vi "Config.vi"() -> ()   [LabVIEW 2020]
uses:
  Global_Variable/A131258.vi
  Database/Global1.vi
  Global_Variable/Global.vi
  <vilib>/Utility/config.llb/NI_LVConfig.lvlib
panel:
  in  "系数":bool
  in  "产品型号":string(combo)
  in  "删除":bool
  in  "确定":bool
  in  "添加":bool
  in  "退出":bool
  in  "更新":bool
  in  "选项卡控件":enum32{"产品参数", "系统参数"}(tab)
  in  "判定框范围":string[][](table)=[["°"], ["N"], ["°"], ["N"], ["°"], ["N"], ["°"], ["N"]]
  in  "工位坐标轴参数":string[][](table)=[["°"], ["N"], ["°"], ["N"], ["mm"], ["N"], ["mm"], ["N"]]
  in  "结果判定参数":string[][](table)=[["N"], ["N"], ["N"], ["N"], ["N"], ["N"], ["N"], ["N"], ["N"]]
  in  "工位滤波":cluster{"启用滤波":bool, "滤波系数":dbl}
  in  "系统参数设置":string[][](table)=[[""], [""], [""], [""]]
  # "磨合台"
types:
  T1 = enum8{"Enabled", "Disabled", "Disabled and Grayed Out"}
  T2 = typedef "NI_LVConfig.lvlib/Config Data RefNum.ctl" = refnum<k1>
  T3 = cluster{"用户编号":string, "用户名":string, "用户密码(密文)":string, "用户权限":string}
  T4 = cluster{"[0]":cluster{dbl, dbl}, "[1]":cluster{dbl, dbl}, "[2]":cluster{dbl, dbl}, "[3]":cluster{dbl, dbl}, "[4]":cluster{dbl, dbl}, "[5]":cluster{dbl, dbl}, "[6]":cluster{dbl, dbl}, "[7]":cluster{dbl, dbl}, "[8]":cluster{dbl, dbl}}
  T5 = cluster{"[0]":cluster{string, dbl, dbl}, "[1]":cluster{string, dbl, dbl}, "[2]":cluster{string, dbl, dbl}, "[3]":cluster{string, dbl, dbl}}
  T6 = cluster{"[0]":cluster{string, dbl, dbl}, "[1]":cluster{string, dbl, dbl}, "[2]":cluster{string, dbl, dbl}, "[3]":cluster{string, dbl, dbl}, "[4]":cluster{string, dbl, dbl}, "[5]":cluster{string, dbl, dbl}, "[6]":cluster{string, dbl, dbl}, "[7]":cluster{string, dbl, dbl}, "[8]":cluster{string, dbl, dbl}, "[9]":cluster{string, dbl, dbl}}
  T7 = cluster{"正向判定X值":cluster{"单位":string, "下限":dbl, "上限":dbl}, "正向判定Y值":cluster{"单位":string, "下限":dbl, "上限":dbl}, "逆向判定X值":cluster{"单位":string, "下限":dbl, "上限":dbl}, "逆向判定Y值":cluster{"单位":string, "下限":dbl, "上限":dbl}}
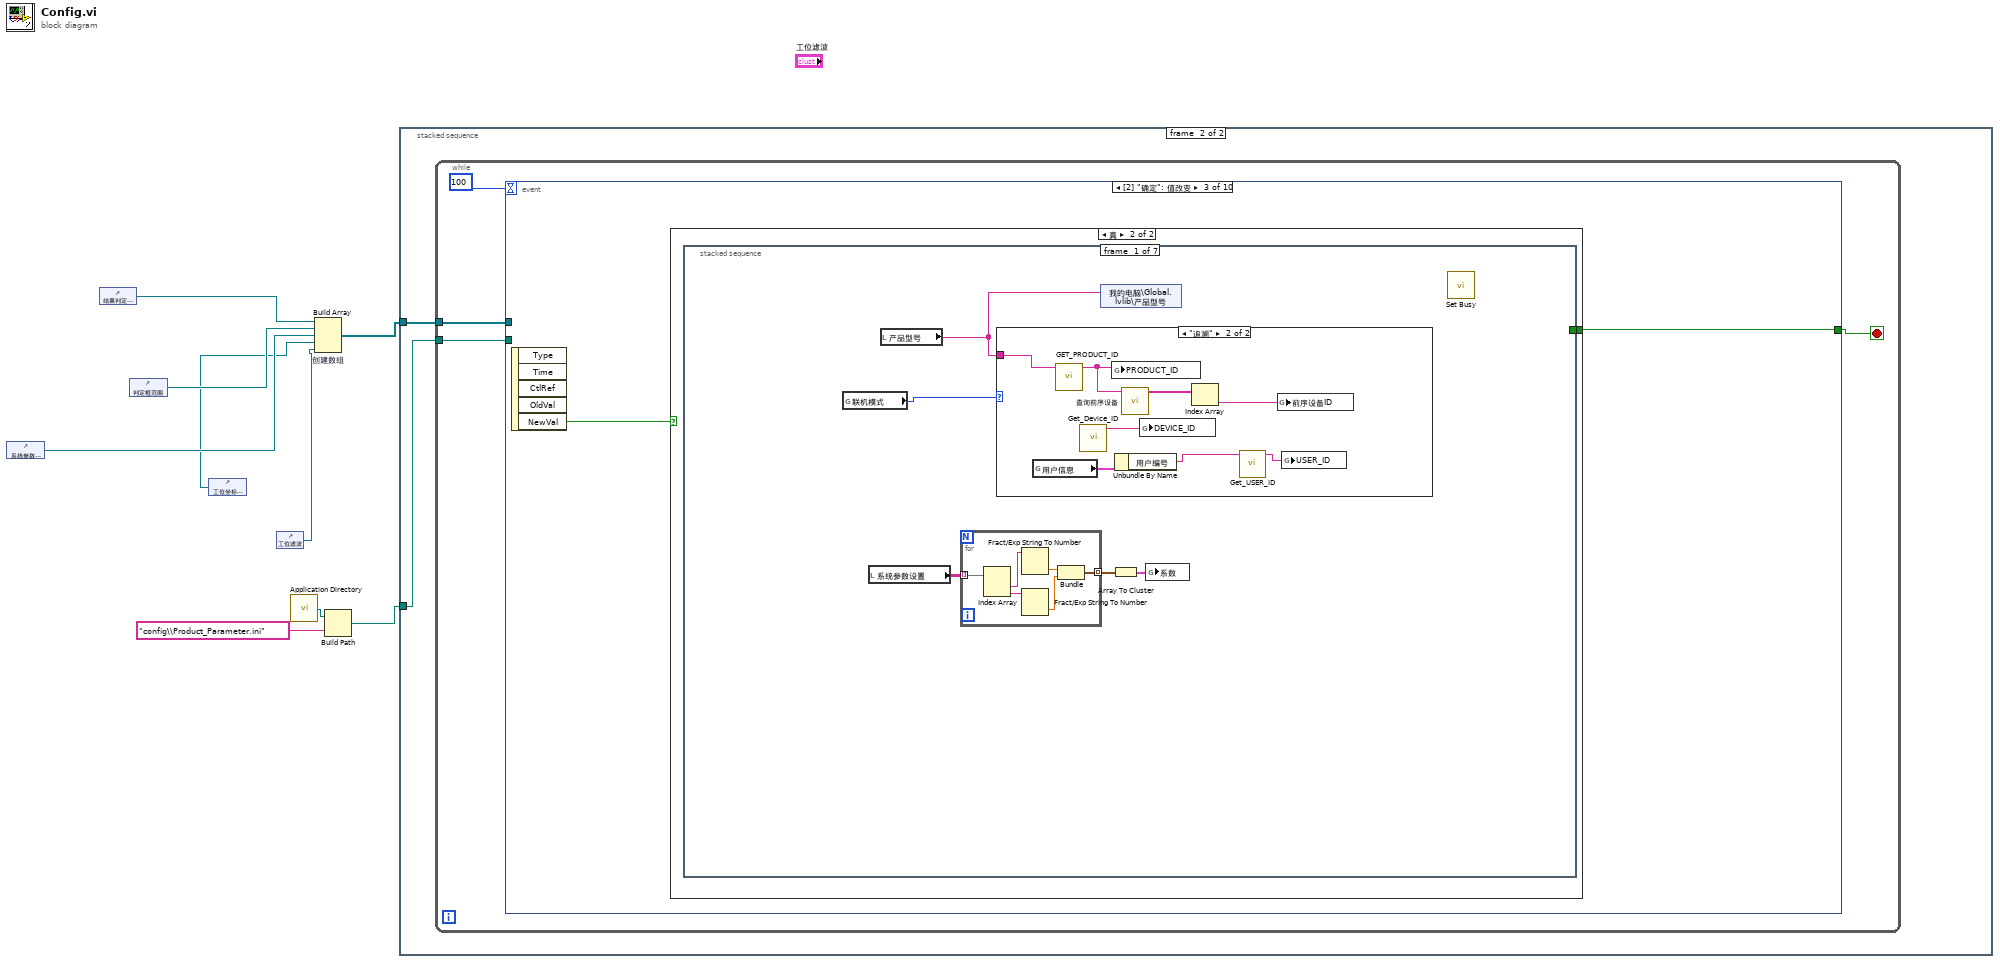
[diagram p0: block diagram]
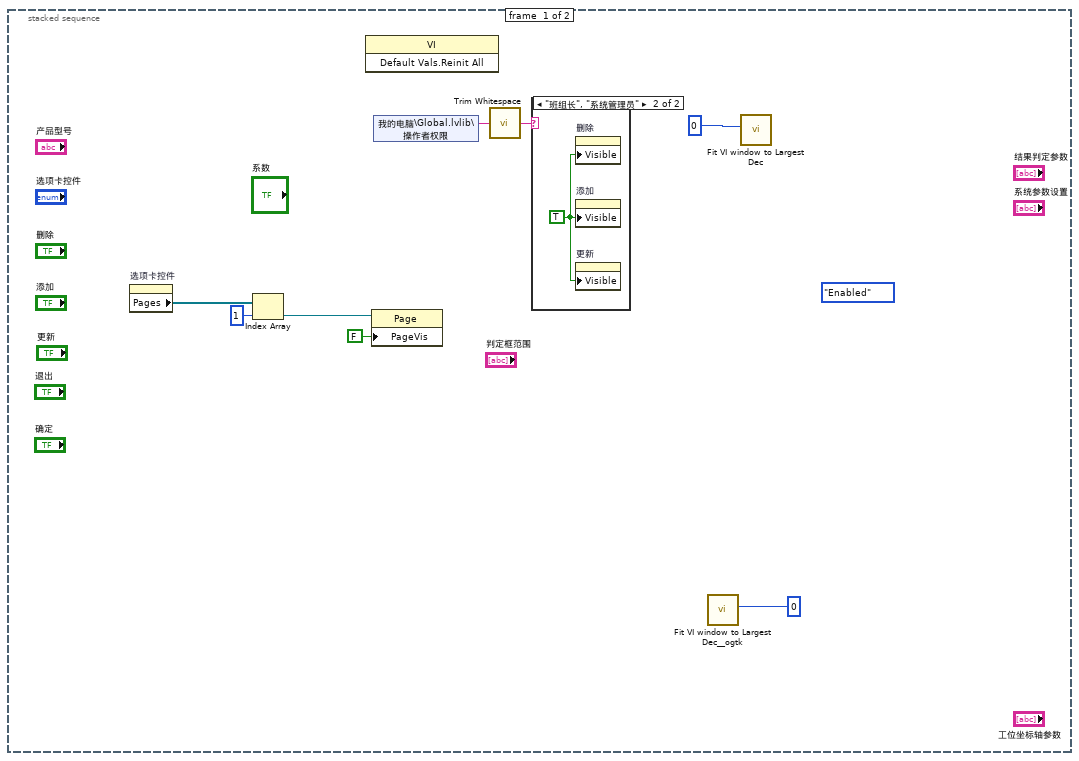
[diagram p2: hidden frame]
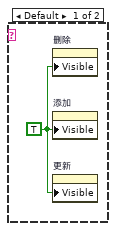
[diagram p3: hidden frame]
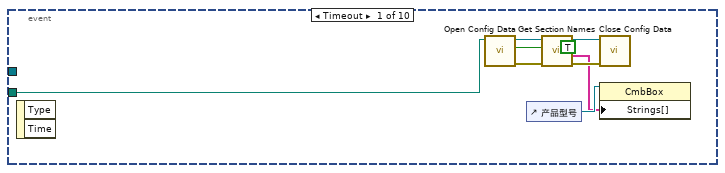
[diagram p4: hidden frame]
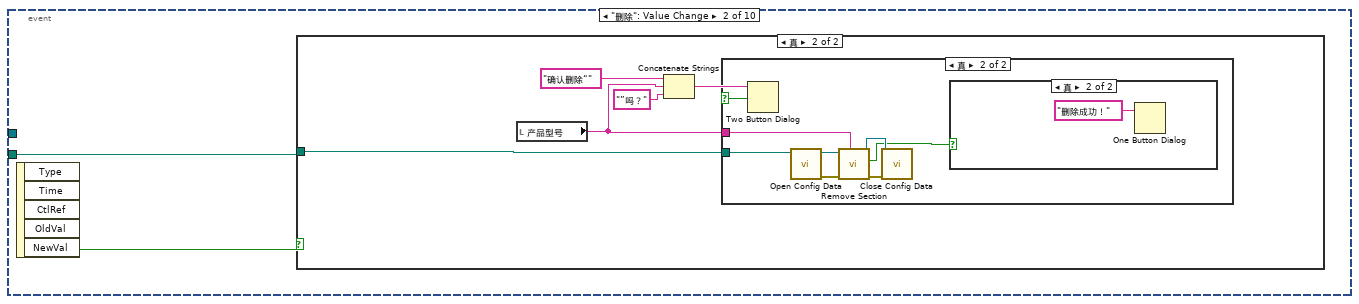
[diagram p5: hidden frame]
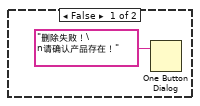
[diagram p8: hidden frame]
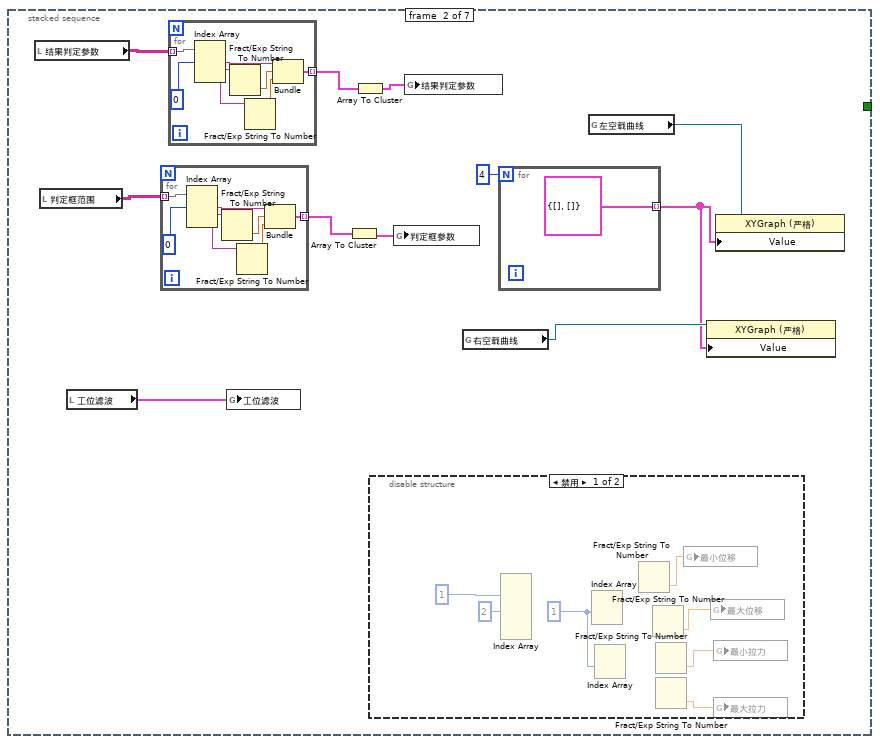
[diagram p11: hidden frame]
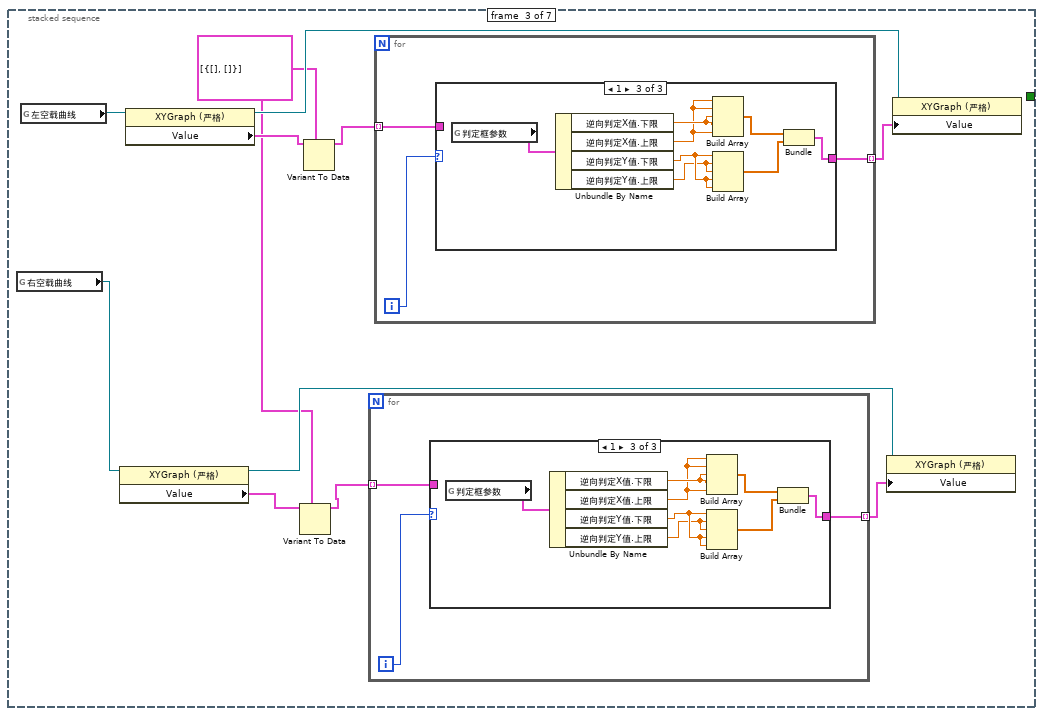
[diagram p13: hidden frame]
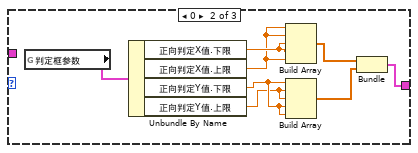
[diagram p15: hidden frame]
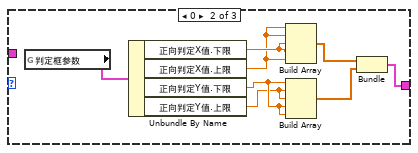
[diagram p17: hidden frame]
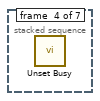
[diagram p18: hidden frame]
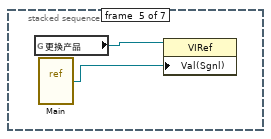
[diagram p19: hidden frame]
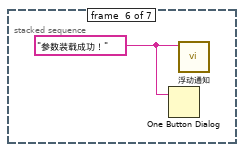
[diagram p20: hidden frame]
diagram:
  n1 = control-ref of="系统参数设置"() -> (w6:refnum<vi>)
  n2 = control-ref of="结果判定参数"() -> (w5:refnum<vi>)
  n3 = control-ref of="判定框范围"() -> (w3:refnum<vi>)
  n4 = control-ref of="工位坐标轴参数"() -> (w2:refnum<vi>)
  n5 = control-ref of="工位滤波"() -> (w1:refnum<vi>)
  n6 = call <vilib>:"Application Directory.vi"() -> ("Application Directory"=w8:path)
  n7 = Build Array "创建数组"(w5, w3, w6, w2, w1) -> (w9:refnum<vi>[])
  n8 = Build Path(base path=w8, name or relative path="config\\Product_Parameter.ini" ("名称或相对路径")) -> (appended path=w7:path)
  n9 = stacked-sequence {
    tunnel: w9 -> [_ w20]
    tunnel: w7 -> [_ w21]
    frame #0 {
      (unwired) T1."Enabled" ("禁用")
      n10 = property on="选项卡控件" class="TabCtl (严格)"() -> ("Pages"=w12:refnum<vi>[])  [unwired: 2 in, 2 out]
      n11 = Index Array(array=w12, index=1 ("索引")) -> (element=w13:refnum<vi>)
      n12 = invoke class="VI" method="Default Vals.Reinit All"() -> ()  [unwired: 3 in, 3 out]
      n13 = property class="Page"(reference=w13, "PageVis"=FALSE ("选项卡可见")) -> ()  [unwired: 1 in, 2 out]
      n14 = shared-variable "我的电脑\\Global.lvlib\\操作者权限"() -> (w17:string)  [unwired: 1 in, 1 out]
      n15 = call <vilib>:"Trim Whitespace.vi"("string"=w17) -> ("trimmed string"=w16:string)  [unwired: 1 in]
      n16 = case shown="\"班组长\", \"系统管理员\"" w16 {
        frame Default {
          w18 = TRUE ("可见")
          n17 = property on="删除" class="Bool (严格)"("Visible"=w18) -> ()  [unwired: 2 in, 2 out]
          n18 = property on="添加" class="Bool (严格)"("Visible"=w18) -> ()  [unwired: 2 in, 2 out]
          n19 = property on="更新" class="Bool (严格)"("Visible"=w18) -> ()  [unwired: 2 in, 2 out]
        }
        frame "班组长", "系统管理员" {
          w19 = TRUE ("可见")
          n20 = property on="删除" class="Bool (严格)"("Visible"=w19) -> ()  [unwired: 2 in, 2 out]
          n21 = property on="添加" class="Bool (严格)"("Visible"=w19) -> ()  [unwired: 2 in, 2 out]
          n22 = property on="更新" class="Bool (严格)"("Visible"=w19) -> ()  [unwired: 2 in, 2 out]
        }
      }
      n23 = call <userlib>:"Fit VI window to Largest Dec__ogtk.vi"("border spacing (2 px)"=0) -> ()  [unwired: 5 in, 2 out]
      n24 = call "Fit VI window to Largest Dec.vi"("border spacing (2 px)"=0) -> ()  [unwired: 5 in, 2 out]
    }
    frame #1 {
      n25 = while {
        tunnel: w21 -> [w25]
        tunnel: w20 -> [w22]
        stop <- w24 stop-if-true
        n26 = event shown="[2] \"确定\": 值改变" {
          selector: _ -> [_ _ _ _ _ _ _ _ _ _]
          dyn-events: _ -> [_ _ _ _ _ _ _ _ _ _]
          timeout: 100 -> [_ _ _ _ _ _ _ _ _ _]
          tunnel: w25 -> [w28 w35 _ w166 w194 _ w217 _ _ _]
          tunnel: [_ _ w51 _ _ TRUE _ _ _ TRUE] -> w24
          tunnel: w22 -> [_ _ _ w164 w192 _ w215 _ _ _]
          event Timeout {
            n27 = event-data() -> ()  [unwired: 1 in, 2 out]
            n28 = call <vilib>:"Open Config Data.vi"("create file if necessary (T)"=TRUE, "configuration file path"=w28) -> ("error out"=w30:errorcluster, "refnum"=w29:T2)  [unwired: 7 in, 1 out]
            n29 = control-ref of="产品型号"() -> (w27:refnum<vi>)
            n30 = call <vilib>:"Get Section Names.vi"("error in (no error)"=w30, "refnum"=w29) -> ("error out"=w32:errorcluster, "section names"=w26:string[], "refnum out"=w31:T2)  [unwired: 7 in]
            n31 = call <vilib>:"Close Config Data.vi"("error in (no error)"=w32, "refnum"=w31) -> ()  [unwired: 8 in, 2 out]
            n32 = property on="属性节点" class="CmbBox"(reference=w27, "Strings[]"=w26) -> ()  [unwired: 1 in, 2 out]
          }
          event "删除": Value Change {
            n33 = event-data() -> ("NewVal"=w34:bool)  [unwired: 1 in, 4 out]
            n34 = case shown="真" w34 {
              tunnel: w35 -> [_ w37]
              frame False {
              }
              frame True {
                n35 = local read "产品型号"() -> (w36:string)
                n36 = Concatenate Strings("确认删除“", w36, "”吗？") -> (w39:string)
                n37 = Two Button Dialog(message=w39) -> (T button?=w38:bool)  [unwired: 2 in]
                n38 = case shown="真" w38 {
                  tunnel: w37 -> [_ w43]
                  tunnel: w36 -> [_ w42]
                  frame False {
                  }
                  frame True {
                    n39 = call <vilib>:"Open Config Data.vi"("configuration file path"=w43) -> ("error out"=w45:errorcluster, "refnum"=w48:T2)  [unwired: 8 in, 1 out]
                    n40 = call <vilib>:"Remove Section.vi"("section"=w42, "error in (no error)"=w45, "refnum"=w48) -> ("error out"=w47:errorcluster, "section exists?"=w44:bool, "refnum out"=w46:T2)  [unwired: 6 in]
                    n41 = call <vilib>:"Close Config Data.vi"("error in (no error)"=w47, "refnum"=w46) -> ()  [unwired: 8 in, 2 out]
                    n42 = case shown="真" w44 {
                      frame False {
                        n43 = One Button Dialog(message="删除失败！\n请确认产品存在！" ("消息")) -> ()  [unwired: 1 in, 1 out]
                      }
                      frame True {
                        n44 = One Button Dialog(message="删除成功！" ("消息")) -> ()  [unwired: 1 in, 1 out]
                      }
                    }
                  }
                }
              }
            }
          }
          event "确定": Value Change {
            n45 = event-data() -> ("NewVal"=w52:bool)  [unwired: 1 in, 4 out]
            n46 = case shown="真" w52 {
              tunnel: [_ w53] -> w51
              frame False {
              }
              frame True {
                n47 = stacked-sequence {
                  tunnel: [_ _ _ _ _ _ TRUE] -> w53
                  frame #0 {
                    n48 = global read "Global1.vi" "联机模式"() -> (w57:enum16{"单机", "追溯"})
                    n49 = local read "系统参数设置"() -> (w56:string[][])
                    n50 = local read "产品型号"() -> (w58:string)
                    n51 = for {
                      tunnel: w56 -> [w64] mode=indexing
                      tunnel: [w61] -> w55 mode=indexing
                      n52 = Index Array(array=w64) -> (element #1=w60:string, element #2=w59:string)  [unwired: 2 in]
                      n53 = Fract/Exp String To Number(string=w60) -> (number=w63:dbl)  [unwired: 3 in, 1 out]
                      n54 = Fract/Exp String To Number(string=w59) -> (number=w62:dbl)  [unwired: 3 in, 1 out]
                      n55 = Bundle(w63, w62) -> (w61:cluster{dbl, dbl})  [unwired: 1 in]
                    }
                    n56 = case shown="\"追溯\"" w57 {
                      tunnel: w58 -> [_ w72]
                      frame "单机", Default {
                      }
                      frame "追溯" {
                        n57 = global read "Global1.vi" "用户信息"() -> (w67:T3)
                        n58 = call "GET_PRODUCT_ID.vi"("PRODFUCT_NAME"=w72) -> ("PRODUCT_ID"=w71:string)  [unwired: 10 in]
                        n59 = call "Get_Device_ID.vi"() -> ("Device_ID"=w68:string)  [unwired: 10 in, 1 out]
                        n60 = global write "追溯Global.vi" "PRODUCT_ID"(w71) -> ()
                        n61 = Unbundle By Name(w67) -> ("用户编号"=w66:string)
                        n62 = call "查询前序设备.vi"("PRODUCT_ID"=w71) -> ("前序工位"=w70:string[])  [unwired: 10 in]
                        n63 = global write "追溯Global.vi" "DEVICE_ID"(w68) -> ()
                        n64 = Index Array(array=w70) -> (element=w69:string)  [unwired: 1 in]
                        n65 = call "Get_USER_ID.vi"("USER_EMPLOYEE_ID"=w66) -> ("USER_ID"=w65:string)  [unwired: 9 in, 1 out]
                        n66 = global write "追溯Global.vi" "前序设备ID"(w69) -> ()
                        n67 = global write "追溯Global.vi" "USER_ID"(w65) -> ()
                      }
                    }
                    n68 = shared-variable "我的电脑\\Global.lvlib\\产品型号"(w58) -> ()  [unwired: 1 in, 1 out]
                    n69 = Array To Cluster(array=w55) -> (cluster=w54:T4)
                    n70 = global write "A131258.vi" "系数"(w54) -> ()
                    n71 = call <vilib>:"Set Busy.vi"() -> ()  [unwired: 10 in, 2 out]
                  }
                  frame #1 {
                    n72 = local read "结果判定参数"() -> (w82:string[][])
                    n73 = local read "判定框范围"() -> (w81:string[][])
                    n74 = local read "工位滤波"() -> (w73:cluster{"启用滤波":bool, "滤波系数":dbl})
                    n75 = for {
                      tunnel: w81 -> [w95] mode=indexing
                      tunnel: [w97] -> w80 mode=indexing
                      n76 = Index Array(array=w95, index #1=0) -> (element #1=w96:string, element #2=w94:string, element #3=w93:string)  [unwired: 2 in]
                      n77 = Fract/Exp String To Number(string=w94) -> (number=w99:dbl)  [unwired: 3 in, 1 out]
                      n78 = Fract/Exp String To Number(string=w93) -> (number=w98:dbl)  [unwired: 3 in, 1 out]
                      n79 = Bundle(w96, w99, w98) -> (w97:cluster{string, dbl, dbl})  [unwired: 1 in]
                    }
                    n80 = for {
                      tunnel: w82 -> [w103] mode=indexing
                      tunnel: [w105] -> w83 mode=indexing
                      n81 = Index Array(array=w103, index #1=0) -> (element #1=w104:string, element #2=w102:string, element #3=w101:string)  [unwired: 2 in]
                      n82 = Fract/Exp String To Number(string=w102) -> (number=w107:dbl)  [unwired: 3 in, 1 out]
                      n83 = Fract/Exp String To Number(string=w101) -> (number=w106:dbl)  [unwired: 3 in, 1 out]
                      n84 = Bundle(w104, w107, w106) -> (w105:cluster{string, dbl, dbl})  [unwired: 1 in]
                    }
                    n85 = global write "A131258.vi" "工位滤波"(w73) -> ()
                    n86 = Array To Cluster(array=w80) -> (cluster=w79:T5)
                    n87 = Array To Cluster(array=w83) -> (cluster=w78:T6)
                    n88 = disable-structure shown="禁用" {
                      frame Disabled {
                        w85 = 1 ("索引")
                        n89 = Index Array(index (row) #1=1 ("索引 (行)"), index (row) #2=2 ("索引 (行)")) -> ()  [unwired: 5 in, 3 out]
                        n90 = Index Array(index #1=w85) -> ()  [unwired: 2 in, 2 out]
                        n91 = Index Array(index #1=w85) -> ()  [unwired: 2 in, 2 out]
                        n92 = Fract/Exp String To Number() -> (number=w90:dbl)  [unwired: 4 in, 1 out]
                        n93 = Fract/Exp String To Number() -> (number=w89:dbl)  [unwired: 4 in, 1 out]
                        n94 = Fract/Exp String To Number() -> (number=w88:dbl)  [unwired: 4 in, 1 out]
                        n95 = Fract/Exp String To Number() -> (number=w87:dbl)  [unwired: 4 in, 1 out]
                        n96 = global write "判定参数.vi" "最小位移"(w90) -> ()
                        n97 = global write "判定参数.vi" "最大位移"(w89) -> ()
                        n98 = global write "判定参数.vi" "最小拉力"(w88) -> ()
                        n99 = global write "判定参数.vi" "最大拉力"(w87) -> ()
                      }
                      frame Enabled {
                      }
                    }
                    n100 = global write "A131258.vi" "判定框参数"(w79) -> ()
                    n101 = global write "A131258.vi" "结果判定参数"(w78) -> ()
                    n102 = global read "A131258.vi" "右空载曲线"() -> (w75:refnum<vi>)
                    n103 = for {
                      N: 4 -> [_]
                      tunnel: [cluster{dbl[], dbl[]} {[], []}] -> w74 mode=indexing
                    }
                    n104 = global read "A131258.vi" "左空载曲线"() -> (w77:refnum<vi>)
                    n105 = property class="XYGraph (严格)"(reference=w75, "Value"=w74) -> ()  [unwired: 1 in, 2 out]
                    n106 = property class="XYGraph (严格)"(reference=w77, "Value"=w74) -> ()  [unwired: 1 in, 2 out]
                  }
                  frame #2 {
                    w111 = cluster{dbl[], dbl[]}[] [{[], []}]
                    n107 = global read "A131258.vi" "右空载曲线"() -> (w108:refnum<vi>)
                    n108 = global read "A131258.vi" "左空载曲线"() -> (w118:refnum<vi>)
                    n109 = property class="XYGraph (严格)"(reference=w108) -> (reference out=w112:refnum<vi>, "Value"=w110:cluster{"Y":dbl[], "Y":dbl[]}[])  [unwired: 1 in, 1 out]
                    n110 = property class="XYGraph (严格)"(reference=w118) -> (reference out=w117:refnum<vi>, "Value"=w115:cluster{"Y":dbl[], "Y":dbl[]}[])  [unwired: 1 in, 1 out]
                    n111 = Variant To Data(type=w111, Variant=w110) -> (data=w109:cluster{dbl[], dbl[]}[])  [unwired: 1 in, 1 out]
                    n112 = Variant To Data(type=w111, Variant=w115) -> (data=w114:cluster{dbl[], dbl[]}[])  [unwired: 1 in, 1 out]
                    n113 = for {
                      tunnel: [w120] -> w113 mode=indexing
                      tunnel: w109 -> [w119] mode=indexing
                      i -> [w121]
                      n114 = case shown="1" w121 {
                        tunnel: [w122 w128 w136] -> w120
                        tunnel: w119 -> [w122 _ _]
                        frame Default {
                        }
                        frame 0 {
                          n115 = global read "A131258.vi" "判定框参数"() -> (w127:T7)
                          n116 = Unbundle By Name(w127) -> ("正向判定X值.下限"=w126:dbl, "正向判定X值.上限"=w125:dbl, "正向判定Y值.下限"=w124:dbl, "正向判定Y值.上限"=w123:dbl)
                          n117 = Build Array(w125, w125, w126, w126, w125) -> (w130:dbl[])
                          n118 = Build Array(w124, w123, w123, w124, w124) -> (w129:dbl[])
                          n119 = Bundle(w130, w129) -> (w128:cluster{dbl[], dbl[]})  [unwired: 1 in]
                        }
                        frame 1 {
                          n120 = global read "A131258.vi" "判定框参数"() -> (w135:T7)
                          n121 = Unbundle By Name(w135) -> ("逆向判定X值.下限"=w134:dbl, "逆向判定X值.上限"=w133:dbl, "逆向判定Y值.下限"=w132:dbl, "逆向判定Y值.上限"=w131:dbl)
                          n122 = Build Array(w133, w133, w134, w134, w133) -> (w138:dbl[])
                          n123 = Build Array(w132, w131, w131, w132, w132) -> (w137:dbl[])
                          n124 = Bundle(w138, w137) -> (w136:cluster{dbl[], dbl[]})  [unwired: 1 in]
                        }
                      }
                    }
                    n125 = for {
                      tunnel: [w140] -> w116 mode=indexing
                      tunnel: w114 -> [w139] mode=indexing
                      i -> [w141]
                      n126 = case shown="1" w141 {
                        tunnel: [w142 w148 w156] -> w140
                        tunnel: w139 -> [w142 _ _]
                        frame Default {
                        }
                        frame 0 {
                          n127 = global read "A131258.vi" "判定框参数"() -> (w147:T7)
                          n128 = Unbundle By Name(w147) -> ("正向判定X值.下限"=w146:dbl, "正向判定X值.上限"=w145:dbl, "正向判定Y值.下限"=w144:dbl, "正向判定Y值.上限"=w143:dbl)
                          n129 = Build Array(w145, w145, w146, w146, w145) -> (w150:dbl[])
                          n130 = Build Array(w144, w143, w143, w144, w144) -> (w149:dbl[])
                          n131 = Bundle(w150, w149) -> (w148:cluster{dbl[], dbl[]})  [unwired: 1 in]
                        }
                        frame 1 {
                          n132 = global read "A131258.vi" "判定框参数"() -> (w155:T7)
                          n133 = Unbundle By Name(w155) -> ("逆向判定X值.下限"=w154:dbl, "逆向判定X值.上限"=w153:dbl, "逆向判定Y值.下限"=w152:dbl, "逆向判定Y值.上限"=w151:dbl)
                          n134 = Build Array(w153, w153, w154, w154, w153) -> (w158:dbl[])
                          n135 = Build Array(w152, w151, w151, w152, w152) -> (w157:dbl[])
                          n136 = Bundle(w158, w157) -> (w156:cluster{dbl[], dbl[]})  [unwired: 1 in]
                        }
                      }
                    }
                    n137 = property class="XYGraph (严格)"(reference=w112, "Value"=w113) -> ()  [unwired: 1 in, 2 out]
                    n138 = property class="XYGraph (严格)"(reference=w117, "Value"=w116) -> ()  [unwired: 1 in, 2 out]
                  }
                  frame #3 {
                    n139 = call <vilib>:"Unset Busy.vi"() -> ()  [unwired: 11 in, 1 out]
                  }
                  frame #4 {
                    n140 = global read "Global.vi" "更换产品"() -> (w160:refnum<vi>)
                    n141 = vi-ref "Main.vi"() -> (w159:refnum<vi>)
                    n142 = property class="VIRef"(reference=w160, "Val(Sgnl)"=w159) -> ()  [unwired: 1 in, 2 out]
                  }
                  frame #5 {
                    w161 = "参数装载成功！" ("消息")
                    n143 = One Button Dialog(message=w161) -> ()  [unwired: 1 in, 1 out]
                    n144 = call "浮动通知.vi"("通知内容"=w161) -> ()  [unwired: 11 in]
                  }
                  frame #6 {
                    n145 = control-ref of="本VI"() -> (w162:refnum<vi>)
                    n146 = invoke class="VI" method="FP.Close"(reference=w162) -> ()  [unwired: 2 in, 3 out]
                  }
                }
              }
            }
          }
          event "添加": Value Change {
            n147 = event-data() -> ("NewVal"=w165:bool)  [unwired: 1 in, 4 out]
            n148 = case shown="真" w165 {
              tunnel: w166 -> [_ w170]
              tunnel: w164 -> [_ w167]
              frame False {
              }
              frame True {
                n149 = call "产品添加提示：用户输入"() -> ("产品型号"=w168:string, "确定"=w169:bool)  [unwired: 17 in, 1 out]
                n150 = case shown="真" w169 {
                  tunnel: w170 -> [_ w173]
                  tunnel: w168 -> [_ w172]
                  tunnel: w167 -> [_ w171]
                  frame False {
                  }
                  frame True {
                    n151 = case shown="默认" w172 {
                      selector: w172 -> [_ w177]
                      tunnel: w173 -> [_ w179]
                      tunnel: w171 -> [_ w175]
                      frame "" {
                        n152 = One Button Dialog(message="产品名称不得为空!" ("text")) -> ()  [unwired: 1 in, 1 out]
                      }
                      frame Default {
                        n153 = property on="产品型号" class="CmbBox"() -> ("Strings[]"=w178:string[])  [unwired: 2 in, 2 out]
                        n154 = Search 1D Array(1D array=w178, element=w177) -> (index of element=w176:i32)  [unwired: 1 in]
                        n155 = case shown="-1" w176 {
                          tunnel: w179 -> [_ w183]
                          tunnel: w177 -> [_ w182]
                          tunnel: w175 -> [_ w181]
                          frame Default {
                            n156 = One Button Dialog(message="产品已存在！" ("消息")) -> ()  [unwired: 1 in, 1 out]
                          }
                          frame -1 {
                            n157 = stacked-sequence {
                              tunnel: w183 -> [w186 _]
                              tunnel: w182 -> [w185 _]
                              tunnel: w181 -> [w184 _]
                              frame #0 {
                                n158 = for {
                                tunnel: w186 -> [w190]
                                tunnel: w185 -> [w187]
                                tunnel: w184 -> [w189] mode=indexing
                                n159 = control-ref of="工位坐标轴参数"() -> ()  [unwired: 1 out]
                                n160 = call "Read_Write ParaINI File.vi"("Mode"=enum16{"Read", "Write"}."Write", "Section"=w187, "Filepath"=w190, "Ctl Refnum"=w189) -> ()  [unwired: 7 in, 1 out]
                                }
                              }
                              frame #1 {
                                n161 = One Button Dialog(message="添加成功！" ("消息")) -> ()  [unwired: 1 in, 1 out]
                              }
                            }
                          }
                        }
                      }
                    }
                  }
                }
              }
            }
          }
          event "产品型号": Value Change {
            n162 = event-data() -> ("NewVal"=w193:string)  [unwired: 1 in, 4 out]
            n163 = stacked-sequence {
              tunnel: w194 -> [_ _ w198]
              tunnel: w193 -> [_ w196 _]
              tunnel: w192 -> [_ _ w197]
              frame #0 {
                n164 = control-ref of="本VI"() -> (w195:refnum<vi>)
                n165 = invoke class="VI" method="Default Vals.Reinit All"(reference=w195) -> ()  [unwired: 2 in, 3 out]
              }
              frame #1 {
                n166 = local write "产品型号"(w196) -> ()
              }
              frame #2 {
                n167 = disable-structure shown="启用" {
                  disable-tunnel: w198 -> [w199 w207]
                  disable-tunnel: w197 -> [_ w208]
                  frame Disabled {
                    n168 = for {
                      tunnel: [w203] -> w200 mode=indexing
                      tunnel: w199 -> [w202]
                      n169 = local read "产品型号"() -> (w201:string)
                      n170 = call "Read_Write ParaINI File.vi"("Mode"=enum16{"Read", "Write"}."Read", "Section"=w201, "Filepath"=w202, "Ctl Refnum"=w203) -> ()  [unwired: 7 in, 1 out]
                    }
                  }
                  frame Enabled {
                    n171 = local read "产品型号"() -> (w209:string)
                    n172 = call <vilib>:"Set Busy.vi"() -> ("error out"=w206:errorcluster)  [unwired: 10 in, 1 out]
                    n173 = call "Read_Write INI File.vi"("Mode"=enum16{"Read", "Write"}."Read", "Section"=w209, "error in"=w206, "Filepath"=w207, "Ctl Refnum"=w208) -> ("error out"=w205:errorcluster)  [unwired: 6 in]
                    n174 = call <vilib>:"Unset Busy.vi"("error in (no error)"=w205) -> ()  [unwired: 10 in, 1 out]
                  }
                }
              }
            }
          }
          event "退出": Value Change {
            n175 = event-data() -> ()  [unwired: 1 in, 5 out]
            n176 = control-ref of="本VI"() -> (w213:refnum<vi>)
            n177 = invoke class="VI" method="FP.Close"(reference=w213) -> (reference out=w211:refnum<vi>, error out=w212:errorcluster)  [unwired: 2 in, 1 out]
            n178 = Close Reference(reference=w211, error in (no error)=w212) -> ()  [unwired: 1 out]
          }
          event "更新": Value Change {
            n179 = event-data() -> ("NewVal"=w216:bool)  [unwired: 1 in, 4 out]
            n180 = case shown="真" w216 {
              tunnel: w217 -> [_ w220]
              tunnel: w215 -> [_ w218]
              frame False {
              }
              frame True {
                n181 = for {
                  tunnel: w220 -> [w227]
                  tunnel: [w226] -> w219
                  tunnel: w218 -> [w225] mode=indexing
                  n182 = local read "产品型号"() -> (w229:string)
                  n183 = call "Read_Write ParaINI File.vi"("Mode"=enum16{"Read", "Write"}."Write", "Section"=w229, "Filepath"=w227, "Ctl Refnum"=w225) -> ("error out"=w226:errorcluster)  [unwired: 7 in]
                }
                n184 = case shown="无错误" w219 {
                  frame No Error {
                    n185 = Wait (ms)(milliseconds to wait=u32 500 ("等待时间（毫秒）")) -> ()  [unwired: 1 out]
                    n186 = One Button Dialog(message="更新成功！" ("通知内容")) -> ()  [unwired: 1 in, 1 out]
                  }
                  frame Error {
                    n187 = Wait (ms)(milliseconds to wait=u32 500 ("等待时间（毫秒）")) -> ()  [unwired: 1 out]
                    n188 = call "浮动通知.vi"("通知内容"="更新失败！") -> ()  [unwired: 11 in]
                  }
                }
              }
            }
          }
          event "系数": Mouse Enter {
            n189 = event-data() -> ()  [unwired: 1 in, 4 out]
            n190 = property on="系数" class="Bool"("Colors [4]"=cluster{u32, u32}[] [{16777216, 16777216}] ("颜色[4]")) -> ()  [unwired: 2 in, 2 out]
          }
          event "系数": Value Change {
            n191 = event-data() -> ("NewVal"=w232:bool)  [unwired: 1 in, 5 out]
            n192 = property on="选项卡控件" class="TabCtl (严格)"() -> ("Pages"=w234:refnum<vi>[])  [unwired: 2 in, 2 out]
            n193 = Index Array(array=w234, index=1 ("索引")) -> (element=w233:refnum<vi>)
            n194 = property class="Page"(reference=w233, "PageVis"=w232) -> ()  [unwired: 1 in, 2 out]
          }
          event Panel Close {
            n195 = event-data() -> ()  [unwired: 1 in, 3 out]
          }
        }
      }
    }
  }
